vi "SortArraysVac.vi"(9 "EnIndicators":refnum<vi>[](array[refnum]), 11 "DIMControSet":refnum<vi>[](array[refnum]), 13 "DIMControlMon out":refnum<vi>[](array[refnum]), 15 "DIMControlMon in":refnum<vi>[](array[refnum]), 17 "DIMControlMon":refnum<vi>[](array[refnum]), 19 "FPIndicator":refnum<vi>[](array[refnum])) -> (8 "Boolean (Strict) (sorted)":refnum<vi>[](array[refnum]), 10 "DIMControSet (sorted)":refnum<vi>[](array[refnum]), 12 "DIMControlMon out (sorted)":refnum<vi>[](array[refnum]), 14 "DIMControlMon in (sorted)":refnum<vi>[](array[refnum]), 16 "DIMControlMon (sorted)":refnum<vi>[](array[refnum]), 18 "FPIndicator sorted":refnum<vi>[](array[refnum]))   [LabVIEW 2014, in "Panels.lvlib"]
uses:
  Panels.lvlib
panel:
  out "EnIndicators  Array":string[](array[string])
  out "EnIndicators Array out":string[](array[string])
  out "DIMControlMon out Array sorted":string[](array[string])
  out "DIMControlMon out Array":string[](array[string])
  out "DIMControlMon Array sorted":string[](array[string])
  out "DIMControSet Array out":string[](array[string])
  out "DIMControlMon in Array sorted":string[](array[string])
  out "FPIndicator Array sorted":string[](array[string])
  out "DIMControSet Array":string[](array[string])
  out "DIMControlMon in Array":string[](array[string])
  out "FPIndicator Array":string[](array[string])
  out "DIMControlMon Array":string[](array[string])
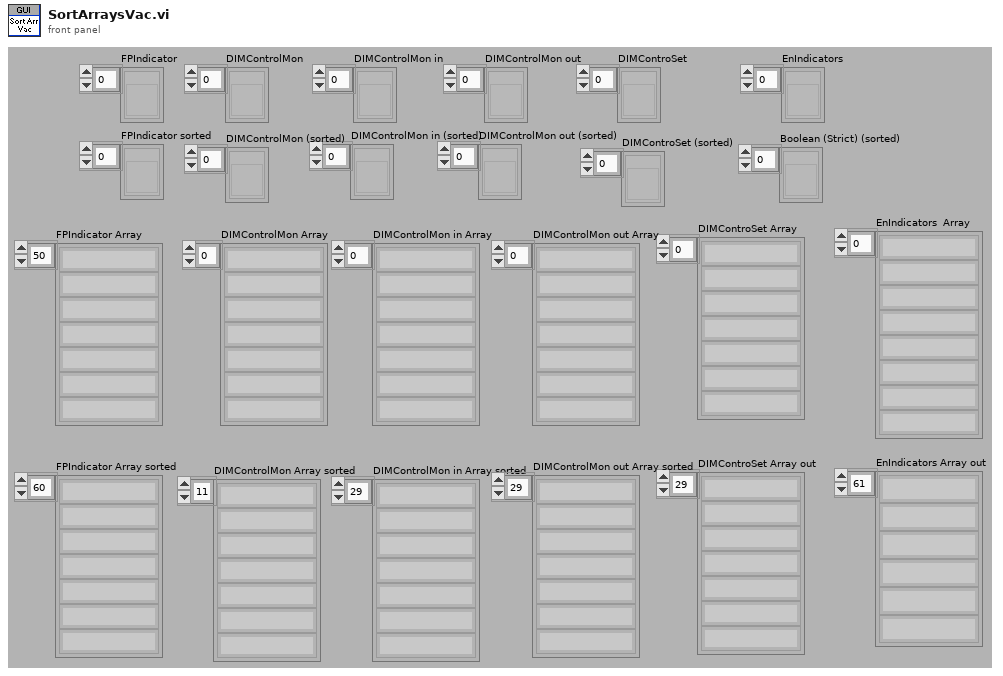
[diagram p1: front panel]
types:
  T1 = enum16{"Boolean", "DigitalNumeric", "DIM-Double", "DIM-Double-Array", "DIM-Short", "Boolean (Strict)"}
  T2 = enum16{"Boolean", "DigitalNumeric", "DIM-Double", "DIM-Double-Array", "DIM-Short"}
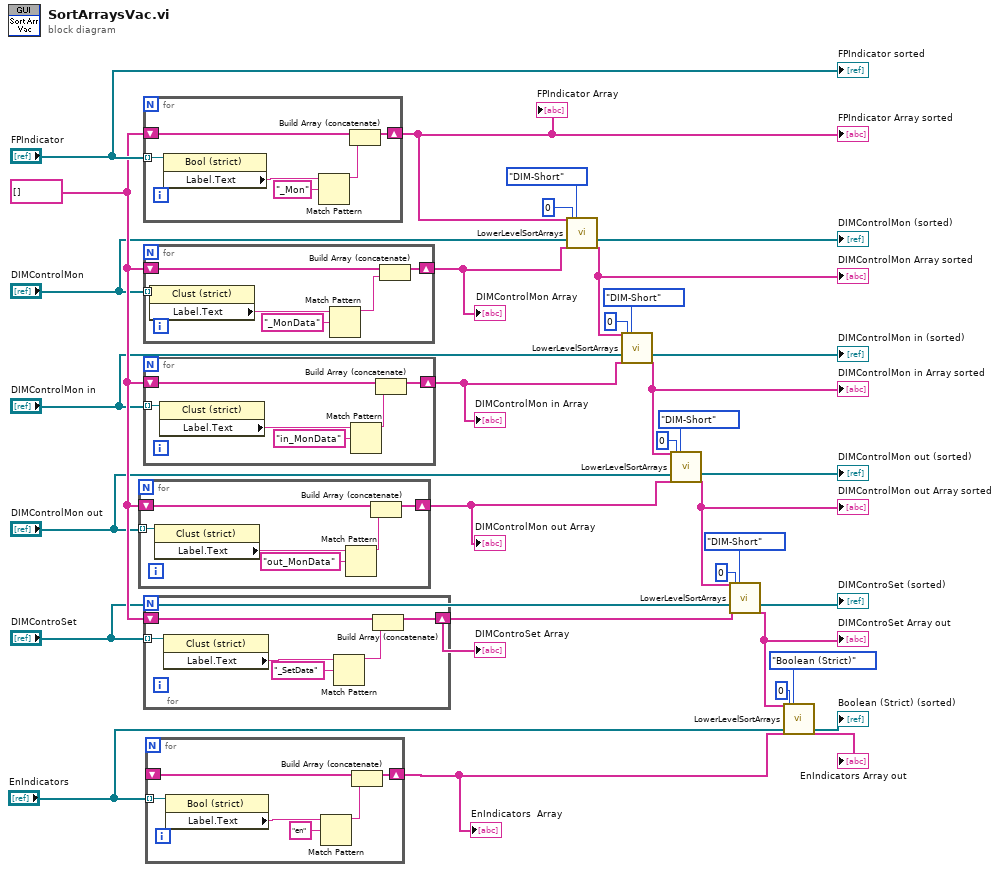
[diagram p0: block diagram]
diagram:
  w22 = string[] []
  n1 = for {
    tunnel: "DIMControlMon out" -> [w37] mode=indexing
    shift-right: [w34] -> w24
    shift-left: w22 -> [w35]
    n2 = property class="Clust (strict)"(reference=w37) -> ("Label.Text"=w38:string)  [unwired: 1 in, 2 out]
    n3 = Match Pattern(string=w38, regular expression="out_MonData") -> (before substring=w36:string)  [unwired: 1 in, 3 out]
    n4 = Build Array (concatenate)(w35, w36) -> (w34:string[])
  }
  "DIMControlMon out Array" <- w24
  n5 = for {
    tunnel: "FPIndicator" -> [w45] mode=indexing
    shift-right: [w40] -> w28
    shift-left: w22 -> [w41]
    n6 = property class="Bool (strict)"(reference=w45) -> ("Label.Text"=w43:string)  [unwired: 1 in, 2 out]
    n7 = Match Pattern(string=w43, regular expression="_Mon") -> (before substring=w42:string)  [unwired: 1 in, 3 out]
    n8 = Build Array (concatenate)(w41, w42) -> (w40:string[])
  }
  "FPIndicator Array" <- w28
  "FPIndicator Array sorted" <- w28
  n9 = for {
    tunnel: "DIMControlMon" -> [w51] mode=indexing
    shift-right: [w50] -> w27
    shift-left: w22 -> [w49]
    n10 = property class="Clust (strict)"(reference=w51) -> ("Label.Text"=w47:string)  [unwired: 1 in, 2 out]
    n11 = Match Pattern(string=w47, regular expression="_MonData") -> (before substring=w46:string)  [unwired: 1 in, 3 out]
    n12 = Build Array (concatenate)(w49, w46) -> (w50:string[])
  }
  "DIMControlMon Array" <- w27
  n13 = for {
    tunnel: "DIMControlMon in" -> [w55] mode=indexing
    shift-right: [w52] -> w33
    shift-left: w22 -> [w53]
    n14 = property class="Clust (strict)"(reference=w55) -> ("Label.Text"=w56:string)  [unwired: 1 in, 2 out]
    n15 = Match Pattern(string=w56, regular expression="in_MonData") -> (before substring=w54:string)  [unwired: 1 in, 3 out]
    n16 = Build Array (concatenate)(w53, w54) -> (w52:string[])
  }
  "DIMControlMon in Array" <- w33
  n17 = for {
    tunnel: "DIMControSet" -> [w61] mode=indexing
    shift-right: [w58] -> w30
    shift-left: w22 -> [w59]
    n18 = property class="Clust (strict)"(reference=w61) -> ("Label.Text"=w62:string)  [unwired: 1 in, 2 out]
    n19 = Match Pattern(string=w62, regular expression="_SetData") -> (before substring=w60:string)  [unwired: 1 in, 3 out]
    n20 = Build Array (concatenate)(w59, w60) -> (w58:string[])
  }
  "DIMControSet Array" <- w30
  n21 = for {
    tunnel: "EnIndicators" -> [w69] mode=indexing
    shift-right: [w64] -> w7
    shift-left: _ -> [w65]
    n22 = property class="Bool (strict)"(reference=w69) -> ("Label.Text"=w67:string)  [unwired: 1 in, 2 out]
    n23 = Match Pattern(string=w67, regular expression="en") -> (before substring=w66:string)  [unwired: 1 in, 3 out]
    n24 = Build Array (concatenate)(w65, w66) -> (w64:string[])
  }
  "EnIndicators  Array" <- w7
  n25 = call "LowerLevelSortArrays.vi"("Sorted Array in"=w28, "DIM-Short"="DIMControlMon", "Unsorted Array in"=w27, "Index"=0, "Type"=T2."DIM-Short") -> ("DIM-Short(sorted)"=→"DIMControlMon (sorted)":refnum<vi>[], "Sorted Array out"=w25:string[])  [unwired: 16 in, 5 out]
  "DIMControlMon Array sorted" <- w25
  n26 = call "LowerLevelSortArrays.vi"("Sorted Array in"=w25, "DIM-Short"="DIMControlMon in", "Unsorted Array in"=w33, "Index"=0, "Type"=T2."DIM-Short") -> ("DIM-Short(sorted)"=→"DIMControlMon in (sorted)":refnum<vi>[], "Sorted Array out"=w21:string[])  [unwired: 16 in, 5 out]
  "DIMControlMon in Array sorted" <- w21
  n27 = call "LowerLevelSortArrays.vi"("Sorted Array in"=w21, "DIM-Short"="DIMControlMon out", "Unsorted Array in"=w24, "Index"=0, "Type"=T2."DIM-Short") -> ("DIM-Short(sorted)"=→"DIMControlMon out (sorted)":refnum<vi>[], "Sorted Array out"=w20:string[])  [unwired: 16 in, 5 out]
  "DIMControlMon out Array sorted" <- w20
  n28 = call "LowerLevelSortArrays.vi"("Sorted Array in"=w20, "DIM-Short"="DIMControSet", "Unsorted Array in"=w30, "Index"=0, "Type"=T2."DIM-Short") -> ("DIM-Short(sorted)"=→"DIMControSet (sorted)":refnum<vi>[], "Sorted Array out"=w6:string[])  [unwired: 16 in, 5 out]
  "DIMControSet Array out" <- w6
  n29 = call "LowerLevelSortArrays.vi"("Sorted Array in"=w6, "Boolean(Strict)"="EnIndicators", "Unsorted Array in"=w7, "Index"=0, "Type"=T1."Boolean (Strict)") -> ("Boolean (Strict) (sorted)"=→"Boolean (Strict) (sorted)":refnum<vi>[], "Sorted Array out"=→"EnIndicators Array out":string[])  [unwired: 16 in, 5 out]
  "FPIndicator sorted" <- "FPIndicator"
